vi "Update Active Attribute Value.vi"(8 "error in (no error)":errorcluster, 10 "Data":variant, 11 "Edit Sequence Dialog in":refnum<class "Sequence Dialog.lvclass">) -> (0 "error out":errorcluster, 3 "Edit Sequence Dialog out":refnum<class "Sequence Dialog.lvclass">)   [LabVIEW 2017, in "Sequence Dialog.lvclass"]
uses:
  <vilib>/gpm_packages/@cs/Test-executive-builder/Source/Test Executive Builder Dialogs/Edit Sequence Dialog/Sequence Dialog.lvclass
  <vilib>/gpm_packages/@cs/Test-executive-builder/Source/Test Executive Builder Dialogs/Edit Sequence Dialog/Sequence Dialog.lvclass/Sequence Dialog.ctl
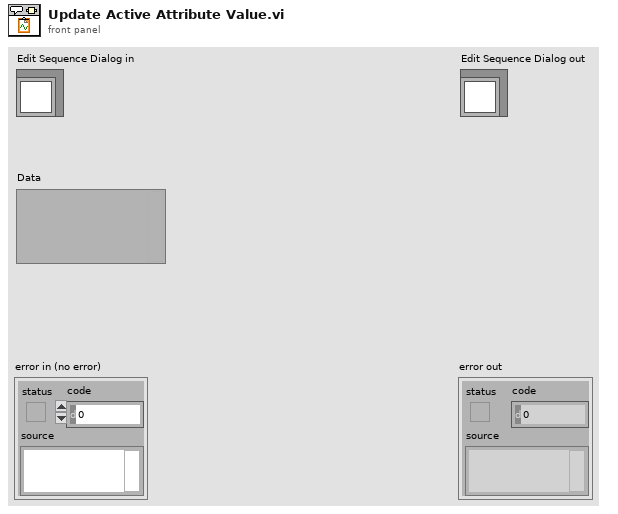
[diagram p1: front panel]
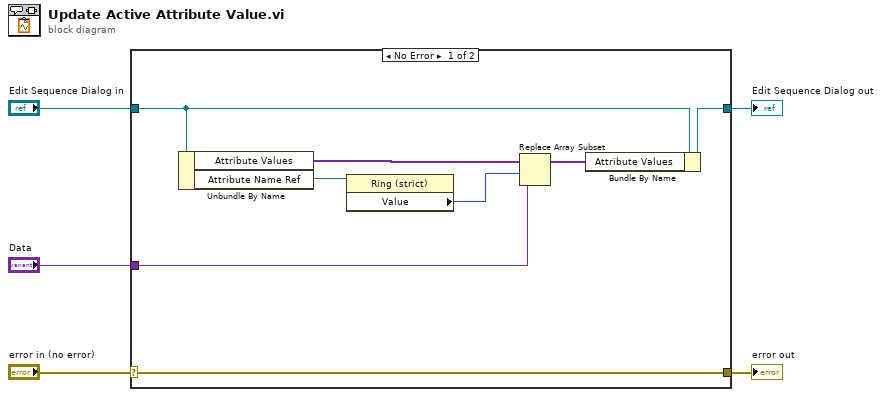
[diagram p0: block diagram]
diagram:
  n1 = case shown="No Error" "error in (no error)" {
    selector: "error in (no error)" -> [w13 w15]
    tunnel: [w13 w15] -> w4
    tunnel: [w7 w14] -> w2
    tunnel: "Edit Sequence Dialog in" -> [w8 w14]
    tunnel: "Data" -> [w9 _]
    frame No Error {
      n2 = Unbundle By Name(w8) -> ("Attribute Values"=w11:variant[], "Attribute Name Ref"=w12:refnum<vi>)
      n3 = property class="Ring (strict)"(reference=w12) -> ("Value"=w10:u16)  [unwired: 1 in, 2 out]
      n4 = Replace Array Subset(array=w11, new element=w9, index=w10) -> (w6:variant[])
      n5 = Bundle By Name(cluster=w8, "Attribute Values"=w6) -> (w7:refnum<class "Sequence Dialog.lvclass">)
    }
    frame Error {
    }
  }
  "error out" <- w4
  "Edit Sequence Dialog out" <- w2
